vi "Print.vi"(8 "error in (no error)":errorcluster, 11 "Message Boolean in":refnum<class "Message Boolean.lvclass">) -> (0 "error out":errorcluster, 2 "String":string, 3 "Message Boolean out":refnum<class "Message Boolean.lvclass">)   [LabVIEW 2016, in "Stream Mediator.lvlib" / "Message Boolean.lvclass"]
doc: "--\nCopyright © 2017 Composed SystemsI All rights reserved.\n\nAuthor: Jon McBee <jon.mcbee@composed.io>\n\nThis library is provided \"AS IS\" ,WITHOUT WARRANTIES OR\nCONDITIONS OF ANY KIND, either express or implied.\n\nComposed Systems -- composed.io\n\nStream 0.0.1.1\nJon McBee - Composed Systems\nCopyright (c) 2017, Composed Systems"
uses:
  <userlib>/Composed Systems/Stream/Mediator/Classes/Message Boolean/Message Boolean.lvclass
  C:/Program Files (x86)/National Instruments/LabVIEW 2016/user.lib/Composed Systems/Stream/Mediator/Classes/Message Interface/Message Interface.lvclass
  <userlib>/Composed Systems/Stream/Mediator/Classes/Message Boolean/Message Boolean.lvclass/Message Boolean.ctl
  <userlib>/Composed Systems/Stream/Mediator/Classes/Message Interface/Message Interface.lvclass
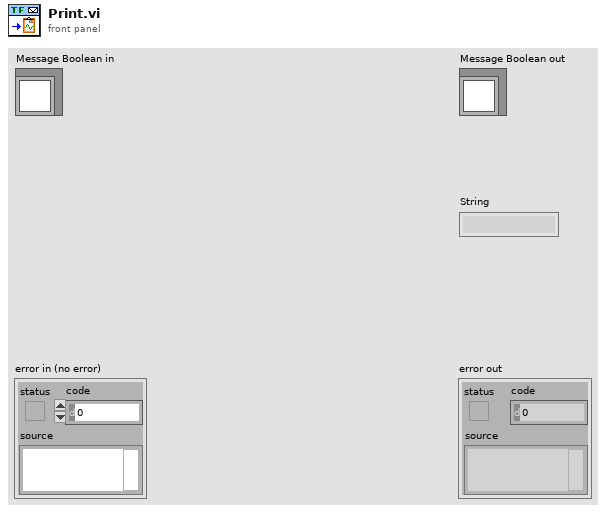
[diagram p1: front panel]
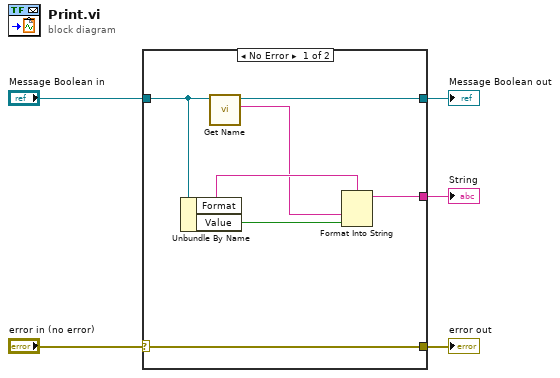
[diagram p0: block diagram]
diagram:
  n1 = case shown="No Error" "error in (no error)" {
    selector: "error in (no error)" -> [w12 w13]
    tunnel: [w12 w13] -> w4
    tunnel: [w11 w14] -> w3
    tunnel: "Message Boolean in" -> [w8 w14]
    tunnel: [w6 _] -> w1
    frame No Error {
      n2 = Unbundle By Name(w8) -> ("Format"=w10:string, "Value"=w9:bool)
      n3 = call <userlib>:"Get Name.vi"("Message Interface in"=w8) -> ("Name"=w7:string, "Message Interface out"=w11:refnum<class "Message Boolean.lvclass">)  [unwired: 8 in, 1 out]
      n4 = Format Into String(format string=w10, w7, w9) -> (resulting string=w6:string)  [unwired: 2 in, 1 out]
    }
    frame Error {
    }
  }
  "error out" <- w4
  "Message Boolean out" <- w3
  "String" <- w1
